vi "i2c.vi"   [LabVIEW 2012, in "Sendmail.lvrbt"]
uses:
  Sendmail.lvrbt
  <vilib>/NXT/Dual Mode Library/Sensors/i2c_sensors.vi
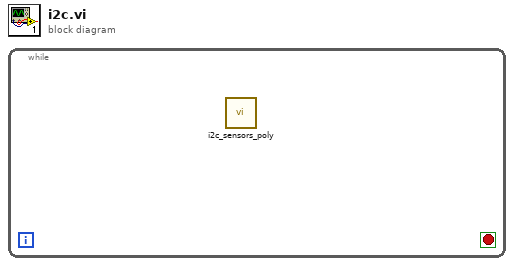
[diagram p0: block diagram]
diagram:
  n1 = while {
    stop <- _ stop-if-true
    n2 = call-poly <vilib>:"i2c_sensors_poly.vi"() -> ()  [unwired: 5 in, 3 out]
  }
